vi "rad_Format Target Information.vi"(7 "System Credentials":T1, 8 "error in":errorcluster, 11 "Targets Information":T2[](array[typedef]) {"Primary NIC"."IP Address Request Mode" items=["Static"=1, "DHCP/Link-Local"=2, "Link-Local Only"=4, "DHCP Only"=8]}) -> (0 "error out":errorcluster, 3 "Targets Information":string[][](array[string]))   [LabVIEW 2020]
uses:
  Target Information.ctl
  subVIs/Targets/TypeDefs/rad_Target Network Settings.ctl
  System Credentials.ctl
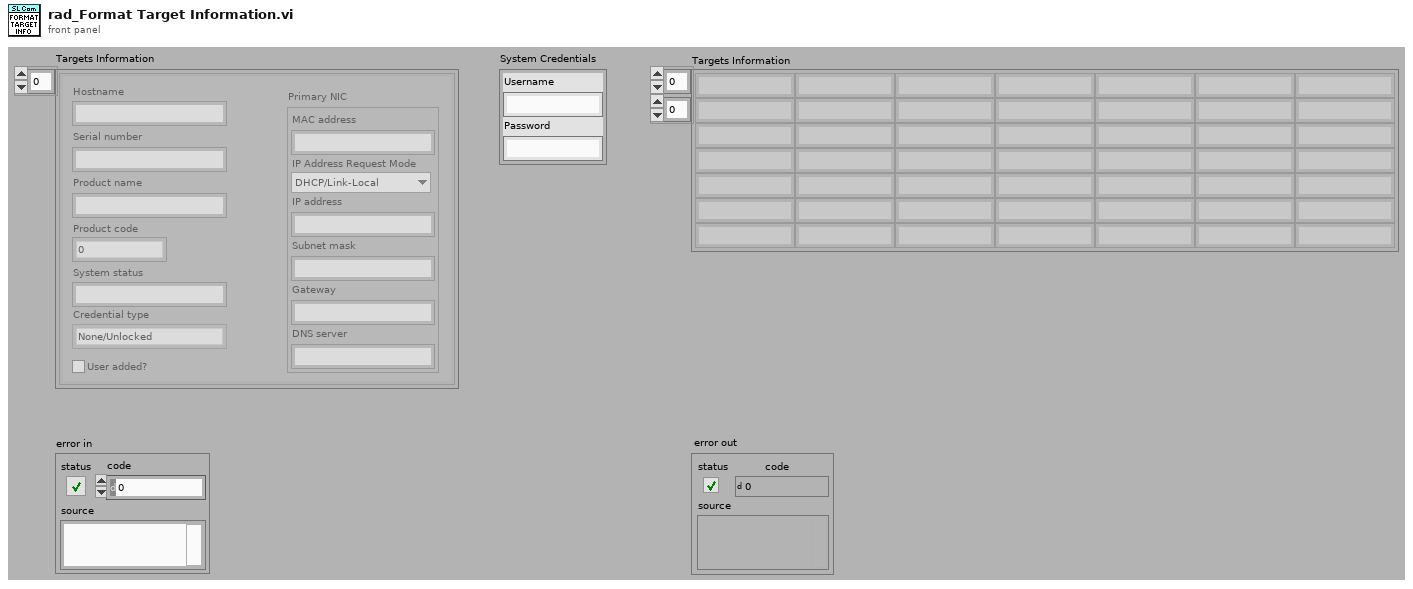
[diagram p1: front panel]
types:
  T1 = typedef "System Credentials.ctl" = cluster{"Username":string, "Password":string}
  T2 = typedef "Target Information.ctl" = cluster{"Hostname":string, "Serial number":string, "Product name":string, "Product code":i32, "System status":string, "Credential type":enum16{"None/Unlocked", "FTP Password", "NIAuth Credentials"}, "User added?":bool, "Primary NIC":T3}
  T3 = typedef "rad_Target Network Settings.ctl" = cluster{"MAC address":string, "IP Address Request Mode":i32, "IP address":string, "Subnet mask":string, "Gateway":string, "DNS server":string}
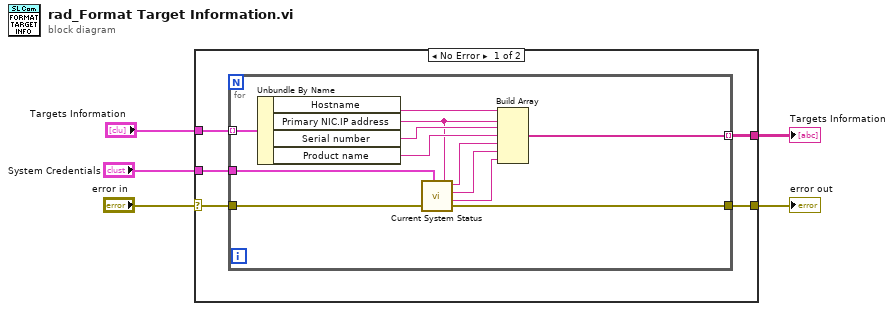
[diagram p0: block diagram]
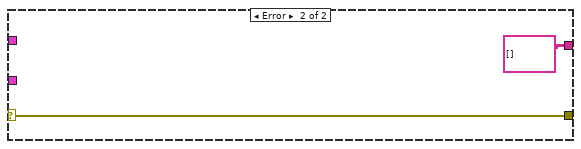
[diagram p2: hidden frame]
diagram:
  n1 = case shown="No Error" "error in" {
    selector: "error in" -> [w7 w24]
    tunnel: [w10 string[][] []] -> w5
    tunnel: "Targets Information" -> [w9 _]
    tunnel: [w8 w24] -> w3
    tunnel: "System Credentials" -> [w6 _]
    frame No Error {
      n2 = for {
        tunnel: w9 -> [w22] mode=indexing
        tunnel: [w19] -> w10 mode=indexing
        tunnel: w7 -> [w16]
        tunnel: [w15] -> w8
        tunnel: w6 -> [w11]
        n3 = Unbundle By Name(w22) -> ("Hostname"=w21:string, "Primary NIC.IP address"=w17:string, "Serial number"=w18:string, "Product name"=w20:string)
        n4 = call "Current System Status.vi"("System Credentials"=w11, "error in"=w16, "IP address"=w17) -> ("error out"=w15:errorcluster, "Requires Update?"=w12:string, "ImageTitle"=w13:string, "Firmware Version"=w14:string)  [unwired: 5 in]
        n5 = Build Array(w21, w17, w18, w20, w14, w13, w12) -> (w19:string[])
      }
    }
    frame Error {
    }
  }
  "Targets Information" <- w5
  "error out" <- w3
